vi "DebbugingOptionsExample.vi"() -> ()   [LabVIEW 2020]
doc: "VI to present debbuging option in LabVIEW. Comments in Polish."
panel:
  out "XY Graph":cluster{dbl[], dbl[]}(graph)
  in  "Value":dbl
  in  "Error In":errorcluster
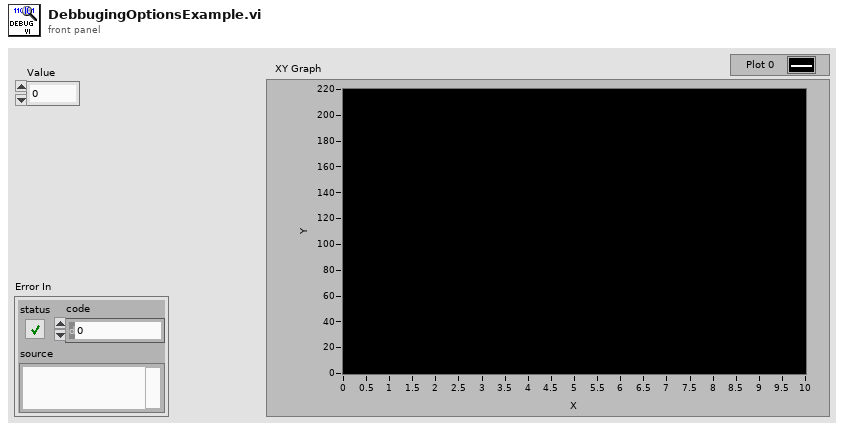
[diagram p1: front panel]
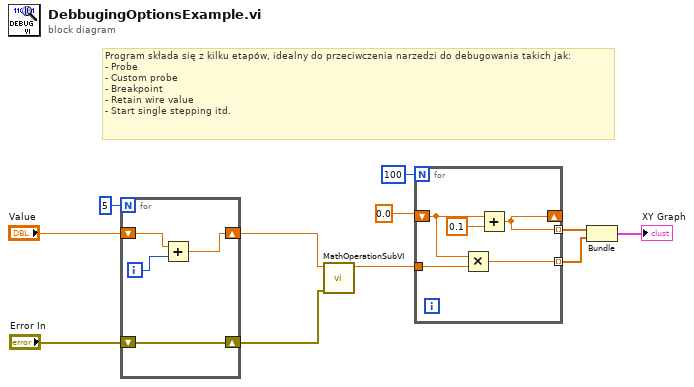
[diagram p0: block diagram]
diagram:
  # "Program składa się z kilku etapów, idealny do przeciwczenia narzedzi do debugowania takich jak:\n- Probe\n- Custom probe\n- Breakpoint\n- Retain wire value \n- Start single stepping itd."
  n1 = for {
    N: 5 -> [_]
    shift-right: [w12] -> w8
    shift-left: "Error In" -> [w12]
    shift-right: [w13] -> w7
    shift-left: "Value" -> [w14]
    i -> [w15]
    n2 = Add(x=w14, y=w15) -> (x+y=w13:dbl)
  }
  n3 = call "MathOperationSubVI.vi"("Error In"=w8, "Main value in"=w7) -> ("Result"=w6:dbl)  [unwired: 8 in, 1 out]
  n4 = for {
    N: 100 -> [_]
    tunnel: w6 -> [w19]
    shift-right: [w17] -> _
    shift-left: 0.0 -> [w20]
    tunnel: [w17] -> w3 mode=indexing
    tunnel: [w18] -> w1 mode=indexing
    n5 = Multiply(x=w20, y=w19) -> (x*y=w18:dbl)
    n6 = Add(x=w20, y=0.1) -> (x+y=w17:dbl)
  }
  n7 = Bundle(w3, w1) -> (→"XY Graph":cluster{dbl[], dbl[]})  [unwired: 1 in]
